vi "MuxSwitchSingle.vi"(7 "MUX address":u32=1 min=1 max=12 step=1, 8 "error in (no error)":errorcluster, 9 "Channel":i32=1 min=1 max=12 step=1, 10 "C1 / C2":i32=1 min=1 max=12 step=1, 11 "LXIPXISwitching in":refnum<class "LXIPXISwitching.lvclass">) -> (0 "error out":errorcluster, 2 "command string":string, 3 "LXIPXISwitching out":refnum<class "LXIPXISwitching.lvclass">)   [LabVIEW 2018, in "LXIPXISwitching.lvclass"]
uses:
  LXIPXISwitching.lvclass
  LXIPXISwitching.lvclass/LXIPXISwitching.ctl
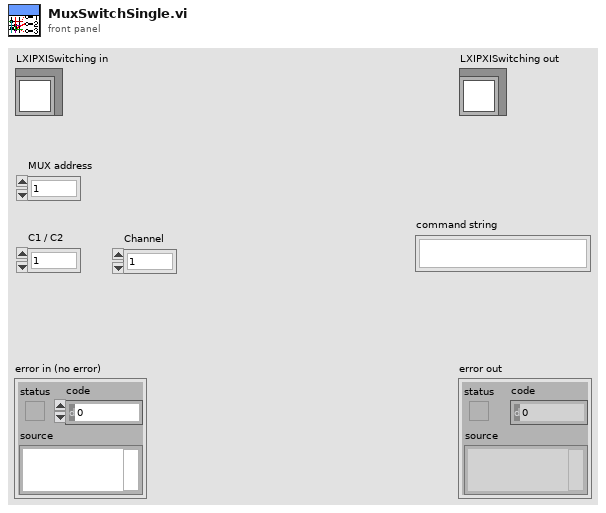
[diagram p1: front panel]
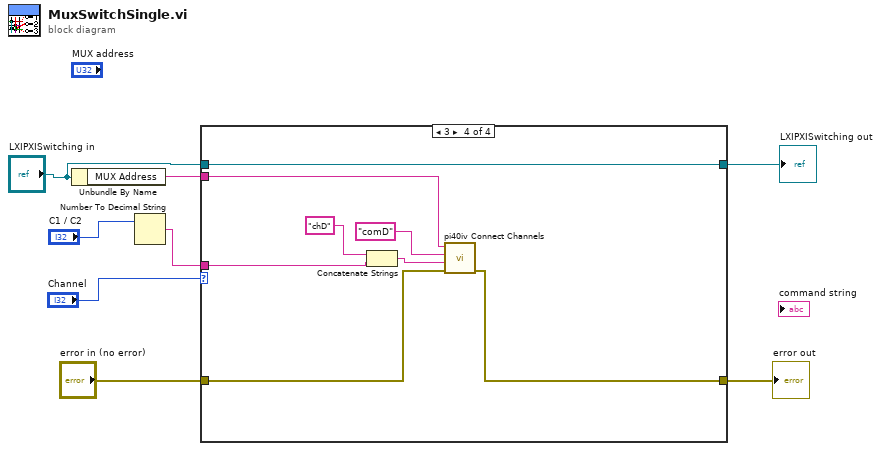
[diagram p0: block diagram]
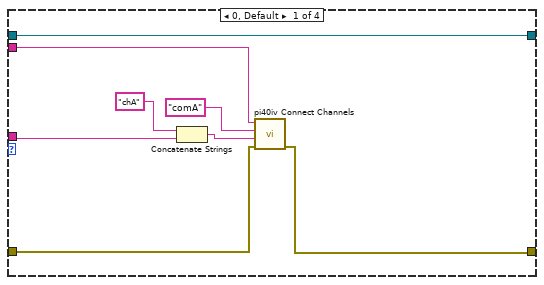
[diagram p2: hidden frame]
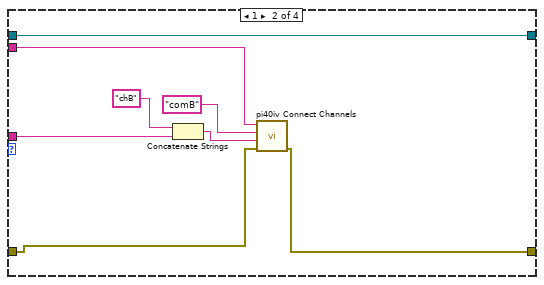
[diagram p3: hidden frame]
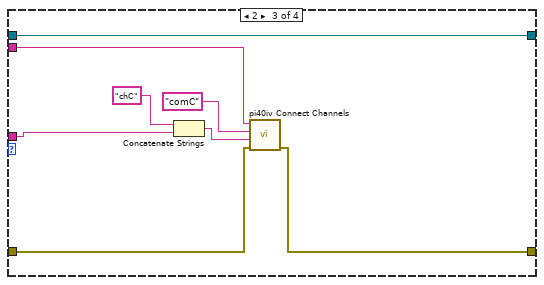
[diagram p4: hidden frame]
diagram:
  n1 = Unbundle By Name("LXIPXISwitching in") -> ("MUX Address"=w3:string)
  n2 = Number To Decimal String(number="C1 / C2") -> (decimal integer string=w6:string)  [unwired: 1 in]
  n3 = case shown="3" "Channel" {
    tunnel: w6 -> [w14 w19 w25 w34]
    tunnel: "error in (no error)" -> [w12 w18 w28 w36]
    tunnel: [w11 w17 w27 w35] -> w4
    tunnel: w3 -> [w10 w20 w26 w33]
    tunnel: "LXIPXISwitching in" -> [w9 w24 w32 w40]
    tunnel: [w9 w24 w32 w40] -> w1
    frame 0, Default {
      n4 = Concatenate Strings("chA" ("string"), w14) -> (w13:string)
      n5 = call <instrlib>:"pi40iv Connect Channels.vi"("error in (no error)"=w12, "channel 2"=w13, "channel 1"="comA", "instrument handle"=w10) -> ("error out"=w11:errorcluster)  [unwired: 6 in, 1 out]
    }
    frame 1 {
      n6 = Concatenate Strings("chB" ("string"), w19) -> (w21:string)
      n7 = call <instrlib>:"pi40iv Connect Channels.vi"("error in (no error)"=w18, "channel 2"=w21, "channel 1"="comB", "instrument handle"=w20) -> ("error out"=w17:errorcluster)  [unwired: 6 in, 1 out]
    }
    frame 2 {
      n8 = Concatenate Strings("chC" ("string"), w25) -> (w29:string)
      n9 = call <instrlib>:"pi40iv Connect Channels.vi"("error in (no error)"=w28, "channel 2"=w29, "channel 1"="comC", "instrument handle"=w26) -> ("error out"=w27:errorcluster)  [unwired: 6 in, 1 out]
    }
    frame 3 {
      n10 = Concatenate Strings("chD" ("string"), w34) -> (w37:string)
      n11 = call <instrlib>:"pi40iv Connect Channels.vi"("error in (no error)"=w36, "channel 2"=w37, "channel 1"="comD", "instrument handle"=w33) -> ("error out"=w35:errorcluster)  [unwired: 6 in, 1 out]
    }
  }
  "error out" <- w4
  "LXIPXISwitching out" <- w1
